vi "CCSetSpecificCharacterSet.vi"(8 "error in (no error)":errorcluster, 11 ".NET Refnum in":refnum<k24>) -> (0 "error out":errorcluster, 3 ".NET Refnum out":refnum<k24>)   [LabVIEW 2013]
uses:
  C:/Users/Simon/SkyDrive/LabView/2013/DM2020/DICOM/ClearCanvasNewBuild/ClearCanvas.Dicom.dll
  ClearCanvasNewBuild/ClearCanvas.Dicom.dll
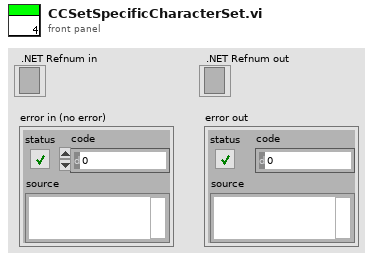
[diagram p1: front panel]
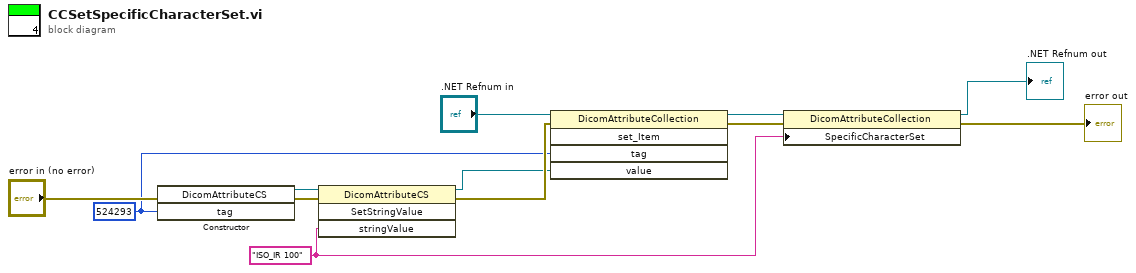
[diagram p0: block diagram]
diagram:
  w10 = 524293
  w1 = "ISO_IR 100" ("stringValue")
  n1 = constructor class="DicomAttributeCS"(error in="error in (no error)", "tag"=w10) -> (reference out=w8:refnum<k24>, error out=w7:errorcluster)  [unwired: 2 in, 2 out]
  n2 = invoke class="DicomAttributeCS" method="SetStringValue"(reference=w8, error in=w7, "stringValue"=w1) -> (reference out=w9:refnum<k24>, error out=w11:errorcluster)  [unwired: 1 in, 2 out]
  n3 = invoke class="DicomAttributeCollection" method="set_Item"(reference=".NET Refnum in", error in=w11, "tag"=w10, "value"=w9) -> (reference out=w5:refnum<k24>, error out=w4:errorcluster)  [unwired: 1 in, 3 out]
  n4 = property class="DicomAttributeCollection"(reference=w5, error in=w4, "SpecificCharacterSet"=w1) -> (reference out=→".NET Refnum out":refnum<k24>, error out=→"error out":errorcluster)
